vi "Overlay.vi"(8 "error in":errorcluster, 10 "Cursor Points":T1[](array[typedef]) {"Y" format="%.2f"; "X" format="%.2f"}, 11 "Refnum in":T2) -> (0 "error out":errorcluster, 3 "Refnum out":T2)   [LabVIEW 2019, in "Andor.lvlib"]
uses:
  Andor.lvlib
  <vilib>/vision/Image Controls.llb/IMAQ Image.ctl
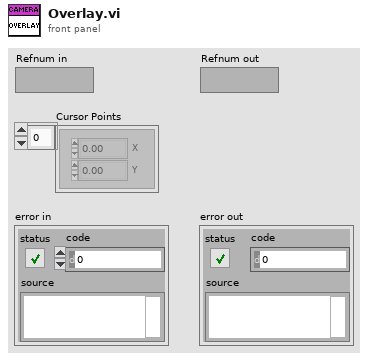
[diagram p1: front panel]
types:
  T1 = typedef "IMAQ Point" = cluster{"X":sgl, "Y":sgl}
  T2 = typedef "IMAQ Image.ctl" = refnum<image>
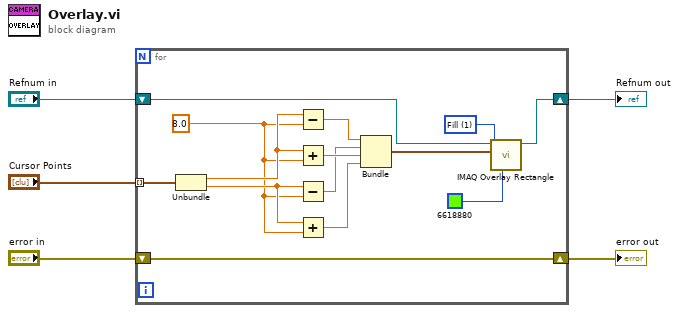
[diagram p0: block diagram]
diagram:
  n1 = for {
    tunnel: "Cursor Points" -> [w17] mode=indexing
    shift-right: [w8] -> w2
    shift-left: "error in" -> [w8]
    shift-right: [w18] -> w5
    shift-left: "Refnum in" -> [w19]
    w6 = sgl 8.0 ("y")
    w9 = u32 1 items=["Frame", "Fill", "Highlight"] ("Drawing Mode (Frame)")
    n2 = Unbundle(w17) -> ("X"=w10:sgl, "Y"=w13:sgl)
    n3 = Subtract(x=w10, y=w6) -> (x-y=w15:sgl)
    n4 = Add(x=w10, y=w6) -> (x+y=w16:sgl)
    n5 = Subtract(x=w13, y=w6) -> (x-y=w12:sgl)
    n6 = Add(x=w13, y=w6) -> (x+y=w14:sgl)
    n7 = Bundle(w15, w12, w16, w14) -> (w11:cluster{sgl, sgl, sgl, sgl})  [unwired: 1 in]
    n8 = call "IMAQ Overlay Rectangle"("Color"=u32 6618880, "Drawing Mode (Frame)"=w9, "Rectangle"=w11, "Image"=w19) -> ("Image Out"=w18:T2)  [unwired: 6 in, 1 out]
  }
  "Refnum out" <- w5
  "error out" <- w2
